vi "GetCoord.vi"(4 "4":bool, 5 "2":bool, 6 "3":bool, 7 "1":bool, 8 "4":i32, 9 "3":i32, 10 "2":i32, 11 "1":i32) -> (2 "OUT":i32)   [LabVIEW 2010]
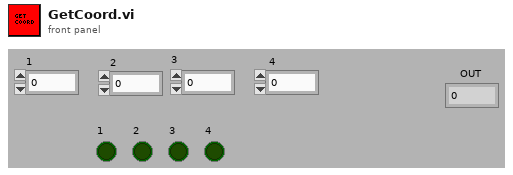
[diagram p1: front panel]
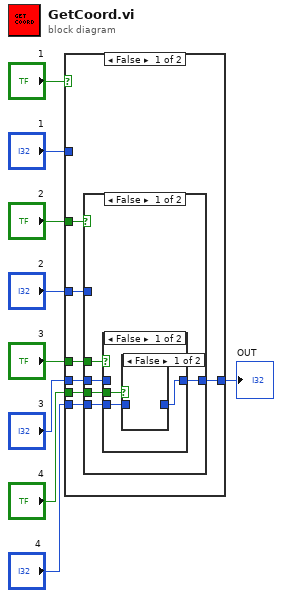
[diagram p0: block diagram]
diagram:
  n1 = case shown="False" "1" {
    tunnel: "1" -> [_ w28]
    tunnel: [w14 w28] -> w7
    tunnel: "2" -> [w16 _]
    tunnel: "2" -> [w15 _]
    tunnel: "3" -> [w13 _]
    tunnel: "3" -> [w12 _]
    tunnel: "4" -> [w11 _]
    tunnel: "4" -> [w10 _]
    frame False {
      n2 = case shown="False" w16 {
        tunnel: w15 -> [_ w27]
        tunnel: [w20 w27] -> w14
        tunnel: w13 -> [w21 _]
        tunnel: w12 -> [w19 _]
        tunnel: w11 -> [w18 _]
        tunnel: w10 -> [w17 _]
        frame False {
          n3 = case shown="False" w21 {
            tunnel: [w23 w26] -> w20
            tunnel: w19 -> [_ w26]
            tunnel: w18 -> [w24 _]
            tunnel: w17 -> [w22 _]
            frame False {
              n4 = case shown="False" w24 {
                tunnel: [_ w25] -> w23
                tunnel: w22 -> [_ w25]
                frame False {
                }
                frame True {
                }
              }
            }
            frame True {
            }
          }
        }
        frame True {
        }
      }
    }
    frame True {
    }
  }
  "OUT" <- w7
